vi "Configured Connection.vi"(8 "error in (no error)":errorcluster, 11 "SerialConfigPanel in":refnum<class "SerialConfigPanel.lvclass">) -> (0 "error out":errorcluster, 2 "Configured Connection":refnum<class "Connection.lvclass">, 3 "SerialConfigPanel out":refnum<class "SerialConfigPanel.lvclass">)   [LabVIEW 2020, in "LV-Term.lvlib" / "SerialConfigPanel.lvclass"]
uses:
  SerialConfigPanel.lvclass
  SerialConfigPanel.lvclass/SerialConfigPanel.ctl
  <vilib>/IlluminatedG/IG Serial Stream/Stream-Serial/Serial Client/Serial Client.lvclass
  C:/Program Files (x86)/National Instruments/LabVIEW 2020/vi.lib/IlluminatedG/lv-stream/Connection/Connection.lvclass
  C:/Program Files (x86)/National Instruments/LabVIEW 2020/vi.lib/IlluminatedG/lv-stream/Endpoint/Endpoint.lvclass
  C:/Program Files (x86)/National Instruments/LabVIEW 2020/vi.lib/IlluminatedG/IG Serial Stream/Stream-Serial/Serial Client/Serial Client.lvclass
  <vilib>/IlluminatedG/lv-stream/Connection/Connection.lvclass
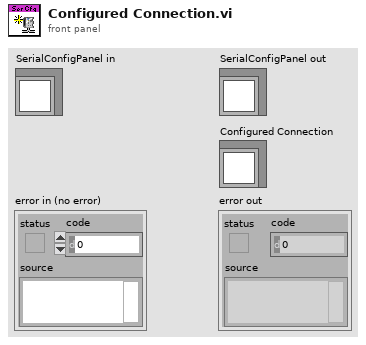
[diagram p1: front panel]
types:
  T1 = typedef "LV-Term.lvlib/SerialConfigPanel.lvclass/Ref Data.ctl" = cluster{"Port":refnum<visa-resource-name>, "Config":T2}
  T2 = typedef "Stream-Serial.lvlib/Serial Client.lvclass/Port Config.ctl" = cluster{"Baud (115200)":u32, "Data Bits (8)":u8, "Stop Bits (1)":T3, "Flow Control":T4, "Use LineTerm?":bool, "LineTerm (\\n)":string, "Timeout ms (10000)":i32, "Parity (None)":T5}
  T3 = typedef "Stream-Serial.lvlib/Serial Client.lvclass/Stop Bits.ctl" = u16
  T4 = typedef "Stream-Serial.lvlib/Serial Client.lvclass/Flow Control.ctl" = u16
  T5 = typedef "Stream-Serial.lvlib/Serial Client.lvclass/Parity.ctl" = enum16{"None", "Odd", "Even", "Mark", "Space"}
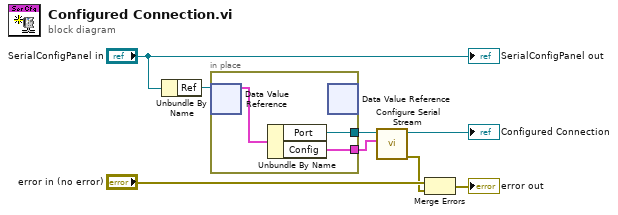
[diagram p0: block diagram]
diagram:
  n1 = Unbundle By Name("SerialConfigPanel in") -> ("Ref"=w7:refnum<data-value>)
  n2 = in-place {
    in-place-border: [w10] -> w4
    in-place-border: [w9] -> w5
    n3 = in-place-dvr #1(w7) -> (w11:T1)  [unwired: 1 out]
    n4 = Unbundle By Name(w11) -> ("Port"=w10:refnum<visa-resource-name>, "Config"=w9:T2)
    n5 = in-place-dvr #1() -> ()  [unwired: 1 in, 2 out]
  }
  n6 = call <vilib>:"Configure Serial Stream.vi"("Port Config (115200 8N1)"=w5, "Serial Port"=w4) -> ("error out"=w2:errorcluster, "Serial Client out"=→"Configured Connection":refnum<class "Serial Client.lvclass">)  [unwired: 8 in]
  n7 = Merge Errors("error in (no error)", w2) -> (→"error out":errorcluster)
  "SerialConfigPanel out" <- "SerialConfigPanel in"
